vi "2Setpoints.vi"   [LabVIEW 2018]
doc: "The myRIO Project template acquires acceleration data from the onboard accelerometer and displays the changes of acceleration values in a waveform chart."
uses:
  <vilib>/platform/TimedLoop/XDataNode/XDataNode.xnode
  <vilib>/Platform/TimedLoop/XDataNode/nitl_modes.ctl
  <vilib>/Platform/TimedLoop/XDataNode/XDNodeRunTimeDep.lvlib
  <vilib>/Platform/TimedLoop/XDataNode/wakeup.ctl
  <vilib>/Platform/TimedLoop/XDataNode/timing_clust.ctl
  <vilib>/myRIO/Common/Instrument Driver Framework/Utilities/typedefs/Generic FPGA Reference.ctl
  <vilib>/myRIO/Common/Instrument Driver Framework/Utilities/typedefs/myRIO v1.0 Reference.ctl
  <vilib>/myRIO/Common/Instrument Driver Framework/Utilities/typedefs/Hardware Version Enum.ctl
  <vilib>/myRIO/Common/Instrument Driver Framework/Utilities/typedefs/myRIO Generic Hardware Reference.ctl
  <vilib>/userdefined/High Color/nirio_resource_hc.ctl
  <vilib>/myRIO/Common/Instrument Driver Framework/myRIO v1.0/Encoder/typedefs/Encoder Channels Enum.ctl
  <vilib>/myRIO/Instrument Drivers/Onboard IO/Encoder/typedefs/Encoder Reference.ctl
  <vilib>/myRIO/Instrument Drivers/Onboard IO/Encoder/Encoder.lvlib
  <vilib>/myRIO/Common/Instrument Driver Framework/myRIO v1.0/Encoder/typedefs/Encoder Signal Mode.ctl
  <vilib>/myRIO/Instrument Drivers/Onboard IO/Encoder/vis/myRIO Encoder Open.xnode
  <vilib>/myRIO/Common/Instrument Driver Framework/myRIO v1.0/Encoder/vis/myRIO v1.1 Open Encoder.vi
  <vilib>/myRIO/Common/Instrument Driver Framework/myRIO v1.0/Encoder/vis/myRIO v1.0 Configure Encoder.vi
  <vilib>/myRIO/Common/Instrument Driver Framework/myRIO v1.0/Encoder/typedefs/Encoder Configuration v1.0.ctl
  <vilib>/myRIO/Instrument Drivers/Onboard IO/PWM/typedefs/PWM Configuration.ctl
  <vilib>/myRIO/Instrument Drivers/Onboard IO/PWM/PWM.lvlib
  <vilib>/myRIO/Common/Instrument Driver Framework/myRIO v1.0/PWM/typedefs/PWM Channels Enum.ctl
  <vilib>/myRIO/Instrument Drivers/Onboard IO/PWM/typedefs/PWM Reference.ctl
  <vilib>/myRIO/Instrument Drivers/Onboard IO/PWM/vis/myRIO PWM Open.xnode
  <vilib>/myRIO/Common/Instrument Driver Framework/myRIO v1.0/PWM/vis/myRIO v1.1 Open PWM.vi
types:
  T1 = typedef "Encoder Signal Mode.ctl" = enum16{"Quadrature phase signal", "Step and direction signal"}
  T2 = typedef "PWM.lvlib/PWM Reference.ctl" = cluster{"myRIO Reference":T3, "PWM Channels Enum":T7, "PWM Configuration":T8}
  T3 = typedef "myRIO Generic Hardware Reference.ctl" = cluster{"myRIO Model":T4, "myRIO Hardware Reference":T5}
  T4 = typedef "Hardware Version Enum.ctl" = enum16{"Unknown", "myRIO-1900", "myRIO-1950", "roboRIO", "NI ELVIS RIO CM", "ELVIS III"}
  T5 = typedef "myRIO v1.0 Reference.ctl" = cluster{"Generic FPGA Reference":T6, "Allow multiple opens":bool}
  T6 = typedef "Generic FPGA Reference.ctl" = refnum<k20>
  T7 = typedef "PWM Channels Enum.ctl" = enum16{"Not Connected", "C/PWM0", "C/PWM1", "A/PWM0", "A/PWM1", "A/PWM2", "A/PWM3", "A/PWM4", "A/PWM5", "A/PWM6", "A/PWM7", "A/PWM8", "A/PWM9", "A/PWM10", "A/PWM11", "A/PWM12", "A/PWM13", "A/PWM14", "A/PWM15", "A/PWM16", "A/PWM17", "A/PWM18", "A/PWM19", "B/PWM0", "B/PWM1", "B/PWM2", "B/PWM3", "B/PWM4", "B/PWM5", "B/PWM6", "B/PWM7", "B/PWM8", "B/PWM9", "B/PWM10", "B/PWM11", "B/PWM12", "B/PWM13", "B/PWM14", "B/PWM15", "B/PWM16", "B/PWM17", "B/PWM18", "B/PWM19", "PWM/PWM0", "PWM/PWM1", "PWM/PWM2", "PWM/PWM3", "PWM/PWM4", "PWM/PWM5", "PWM/PWM6", "PWM/PWM7", "PWM/PWM8", "PWM/PWM9"}
  T8 = typedef "PWM.lvlib/PWM Configuration.ctl" = cluster{"Frequency":dbl, "Duty Cycle":dbl}
  T9 = typedef "Encoder.lvlib/Encoder Reference.ctl" = cluster{"myRIO Reference":T3, "Encoder Channels Enum":T10}
  T10 = typedef "Encoder Channels Enum.ctl" = enum16{"Not Connected", "C/ENC0", "C/ENC1", "A/ENC", "A/ENC0", "A/ENC1", "A/ENC2", "A/ENC3", "A/ENC4", "A/ENC5", "A/ENC6", "A/ENC7", "A/ENC8", "A/ENC9", "B/ENC", "B/ENC0", "B/ENC1", "B/ENC2", "B/ENC3", "B/ENC4", "B/ENC5", "B/ENC6", "B/ENC7", "B/ENC8", "B/ENC9", "DIO/ENC0", "DIO/ENC1", "DIO/ENC2", "DIO/ENC3", "DIO/ENC4"}
  T11 = typedef "XDNodeRunTimeDep.lvlib/timing_clust.ctl" = cluster{"Expected End [f-1]":u64, "Actual End [f-1]":u64, "Finished Late? [f-1]":bool, "Expected End [i-1]":u64, "Actual End [i-1]":u64, "Finished Late? [i-1]":bool, "Expected Start [i]":u64, "Actual Start [i]":u64, "Expected Start [f]":u64, "Actual Start [f]":u64, "Source Name":string, "Structure Name":string, "Period":i64, "Deadline":i64, "Offset":i64, "Start":i64, "Priority":i32, "Timeout":i32, "Mode":T12, "Wakeup Reason":T13, "Error":errorcluster, "Source Type":string, "Secondary Source Type":string, "Global End Time":u64, "Global Start Time":u64, "Frame Duration":u64, "Iteration Duration":u64, "Assigned CPU":i32, "I/O Scan Engine Mode":u32}
  T12 = typedef "XDNodeRunTimeDep.lvlib/nitl_modes.ctl" = enum32{"No Change", "Process missed periods, maintain original phase", "Discard missed periods, maintain original phase", "Process missed periods, ignore original phase", "Discard missed periods, ignore original phase"}
  T13 = typedef "XDNodeRunTimeDep.lvlib/wakeup.ctl" = enum32{"Normal", "Aborted", "Asynchronous wakeup", "Timing source error", "Timed loop error", "Timeout"}
  T14 = cluster{"Double":dbl, dbl, dbl, "seconds since 1Jan1904":timestamp, "Double":dbl, dbl, dbl}
  T15 = cluster{"Double":dbl, "dbl Scaled Value":dbl, "Output":dbl, "seconds since 1Jan1904":timestamp, dbl, dbl, dbl}
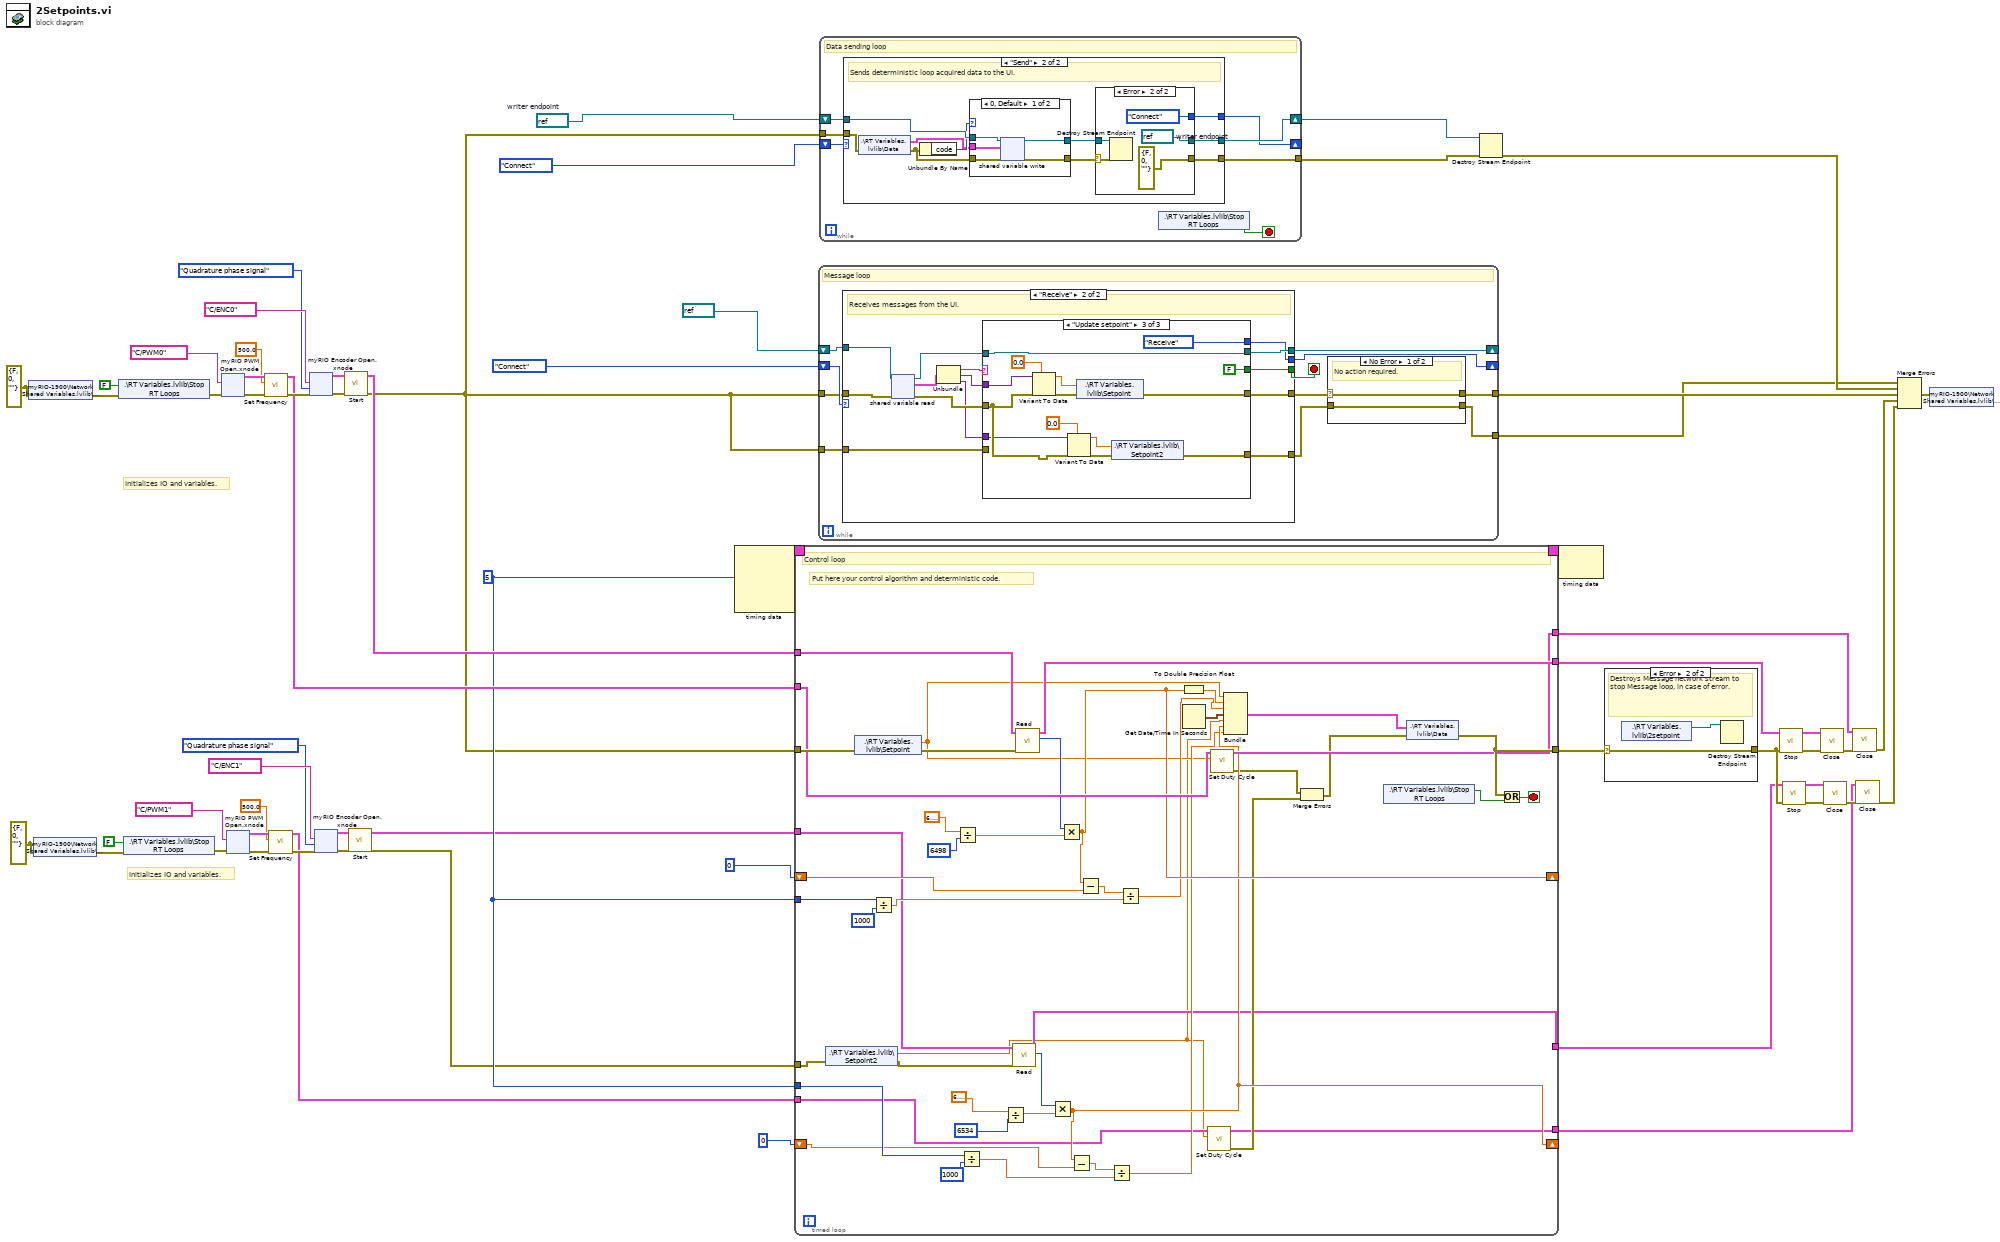
[diagram p0: block diagram]
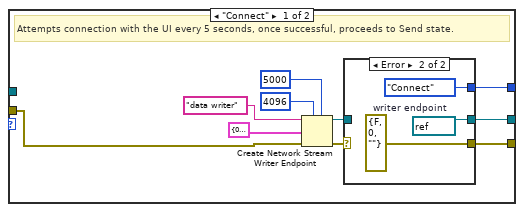
[diagram p3: hidden frame]
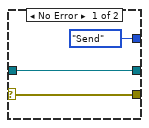
[diagram p4: hidden frame]
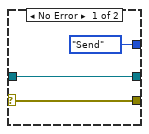
[diagram p5: hidden frame]
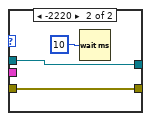
[diagram p6: hidden frame]
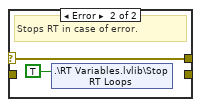
[diagram p7: hidden frame]
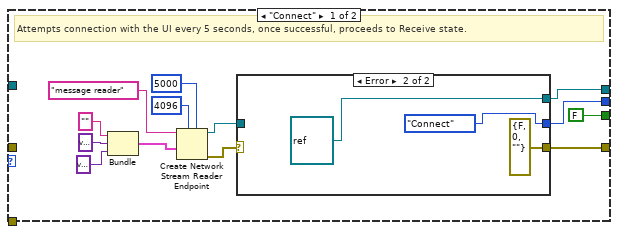
[diagram p8: hidden frame]
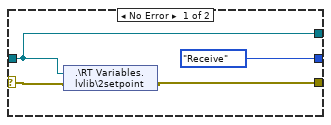
[diagram p9: hidden frame]
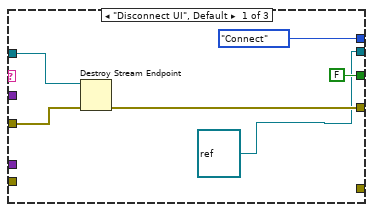
[diagram p10: hidden frame]
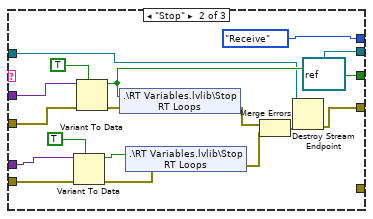
[diagram p11: hidden frame]
diagram:
  w11 = refnum<k21> refnum  # writer endpoint
  w26 = errorcluster {"status"=FALSE, "code"=0, "source"=""} ("error IO")
  w29 = i64 5 ("Period")
  w50 = errorcluster {"status"=FALSE, "code"=0, "source"=""} ("error IO")
  # "Initializes IO and variables."
  # "Initializes IO and variables."
  n1 = shared-variable "myRIO-1900\\Network Shared Variables.lvlib\\error IO"(w50, error in=w50) -> (error out=w51:errorcluster)
  n2 = shared-variable "myRIO-1900\\Network Shared Variables.lvlib\\error IO"(w26, error in=w26) -> (error out=w27:errorcluster)
  n3 = shared-variable ".\\RT Variables.lvlib\\Stop RT Loops"(FALSE ("Stop RT Loops"), error in=w51) -> (error out=w38:errorcluster)
  n4 = shared-variable ".\\RT Variables.lvlib\\Stop RT Loops"(FALSE ("Stop RT Loops"), error in=w27) -> (error out=w19:errorcluster)
  n5 = xnode "myRIO PWM Open.xnode"("error in (no error)"=w38, "Channel Name"=tag "C/PWM0") -> ("error out"=w40:errorcluster, "PWM Ref Out"=w39:T2)  [unwired: 1 in]
  n6 = xnode "myRIO PWM Open.xnode"("error in (no error)"=w19, "Channel Name"=tag "C/PWM1") -> ("error out"=w21:errorcluster, "PWM Ref Out"=w20:T2)  [unwired: 1 in]
  n7 = call <vilib>:"Set Frequency.vi"("error in (no error)"=w40, "Frequency [Hz]"=500.0, "PWM Ref In"=w39) -> ("error out"=w37:errorcluster, "PWM Ref Out"=w34:T2)  [unwired: 6 in]
  n8 = call <vilib>:"Set Frequency.vi"("error in (no error)"=w21, "Frequency [Hz]"=500.0, "PWM Ref In"=w20) -> ("error out"=w18:errorcluster, "PWM Ref Out"=w13:T2)  [unwired: 6 in]
  n9 = xnode "myRIO Encoder Open.xnode"("error in (no error)"=w37, "Channel Name"=tag "C/ENC0", "Encoder Signal Mode"=Encoder_Signal_Mode."Quadrature phase signal") -> ("error out"=w47:errorcluster, "Encoder Ref Out"=w46:T9)  [unwired: 2 in]
  n10 = xnode "myRIO Encoder Open.xnode"("error in (no error)"=w18, "Channel Name"=tag "C/ENC1", "Encoder Signal Mode"=Encoder_Signal_Mode."Quadrature phase signal") -> ("error out"=w24:errorcluster, "Encoder Ref Out"=w23:T9)  [unwired: 2 in]
  n11 = call <vilib>:"Start.vi"("error in (no error)"=w47, "Encoder Ref In"=w46) -> ("error out"=w1:errorcluster, "Encoder Ref Out"=w44:T9)  [unwired: 8 in]
  n12 = call <vilib>:"Start.vi"("error in (no error)"=w24, "Encoder Ref In"=w23) -> ("error out"=w15:errorcluster, "Encoder Ref Out"=w14:T9)  [unwired: 8 in]
  n13 = node-c288(w29) -> (w61:T11)  [unwired: 3 in]
  n14 = timed-loop {
    timing: w61 -> [_]
    timing-out: [_] -> w60
    tunnel: w1 -> [w105]
    tunnel: [w101] -> w49
    tunnel: w44 -> [w100]
    tunnel: [w99] -> w41
    tunnel: w34 -> [w98]
    tunnel: [w96] -> w33
    shift-right: [w90] -> _
    shift-left: 0 -> [w89]
    tunnel: w29 -> [w86]
    shift-right: [w73] -> _
    shift-left: 0 -> [w78]
    tunnel: w29 -> [w79]
    tunnel: w15 -> [w64]
    tunnel: w14 -> [w75]
    tunnel: w13 -> [w71]
    tunnel: [w66] -> w6
    tunnel: [w65] -> w5
    stop <- w102 stop-if-true
    # "Put here your control algorithm and deterministic code."
    # "Control loop"
    n15 = shared-variable ".\\RT Variables.lvlib\\Setpoint2"(error in=w64) -> (w62:dbl, error out=w63:errorcluster)
    n16 = shared-variable ".\\RT Variables.lvlib\\Setpoint"(error in=w105) -> (w67:dbl, error out=w106:errorcluster)
    n17 = Divide(x=w86, y=1000) -> (x/y=w84:dbl)
    n18 = Divide(x=6.283185307179586, y=6498) -> (x/y=w91:dbl)
    n19 = Divide(x=w79, y=1000) -> (x/y=w74:dbl)
    n20 = Divide(x=6.283185307179586, y=6534) -> (x/y=w76:dbl)
    n21 = call <vilib>:"Read.vi"("error in (no error)"=w63, "Encoder Ref In"=w75) -> ("Counter Value"=w77:i32, "Encoder Ref Out"=w66:T9)  [unwired: 5 in, 3 out]
    n22 = call <vilib>:"Read.vi"("error in (no error)"=w106, "Encoder Ref In"=w100) -> ("Counter Value"=w92:i32, "Encoder Ref Out"=w99:T9)  [unwired: 5 in, 3 out]
    n23 = Multiply(x=w77, y=w76) -> (x*y=w73:dbl)
    n24 = Multiply(x=w92, y=w91) -> (x*y=w90:dbl)
    n25 = Subtract(x=w73, y=w78) -> (x-y=w80:dbl)
    n26 = Subtract(x=w90, y=w89) -> (x-y=w88:dbl)
    n27 = Divide(x=w80, y=w74) -> (x/y=w72:dbl)
    n28 = Divide(x=w88, y=w84) -> (x/y=w87:dbl)
    n29 = To Double Precision Float(number=w90) -> (double precision float=w97:dbl)
    n30 = Get Date/Time In Seconds() -> (seconds since 1Jan1904=w104:timestamp)
    n31 = call <vilib>:"Set Duty Cycle.vi"("Duty Cycle"=w62, "PWM Ref In"=w71) -> ("error out"=w70:errorcluster, "PWM Ref Out"=w65:T2)  [unwired: 7 in]
    n32 = call <vilib>:"Set Duty Cycle.vi"("Duty Cycle"=w67, "PWM Ref In"=w98) -> ("error out"=w69:errorcluster, "PWM Ref Out"=w96:T2)  [unwired: 7 in]
    n33 = Bundle("Double"=w67, w97, w87, "seconds since 1Jan1904"=w104, "Double"=w62, w73, w72) -> (w95:T14)  [unwired: 1 in]
    n34 = Merge Errors(w69, w70) -> (w68:errorcluster)
    n35 = shared-variable ".\\RT Variables.lvlib\\Stop RT Loops"() -> (w103:bool)  [unwired: 1 in, 1 out]
    n36 = shared-variable ".\\RT Variables.lvlib\\Data"(w95, error in=w68) -> (error out=w101:errorcluster)
    n37 = Or(x=w101, y=w103) -> (x .or. y?=w102:bool)
  }
  n38 = while {
    tunnel: [w113] -> w53
    shift-right: [w118] -> _
    shift-left: refnum<k21> refnum ("reader endpoint") -> [w116]
    shift-right: [w117] -> _
    shift-left: enum16{"Connect", "Receive"}."Connect" ("Message states") -> [w119]
    tunnel: w1 -> [w115]
    tunnel: [w111] -> w3
    tunnel: w1 -> [w109]
    stop <- w110 stop-if-true
    # "Message loop"
    n39 = case shown="\"Receive\"" w119 {
      tunnel: [w127 w153] -> w114
      tunnel: [w125 w154] -> w118
      tunnel: [w134 w150] -> w117
      tunnel: w116 -> [_ w148]
      tunnel: w115 -> [_ w152]
      tunnel: [FALSE ("Stop RT Loops") w151] -> w110
      tunnel: [_ w145] -> w112
      tunnel: w109 -> [_ w144]
      frame "Connect" {
        # "Attempts connection with the UI every 5 seconds, once successful, proceeds to Receive state."
        n40 = Bundle("", variant, variant) -> (w130:cluster{string, variant, variant})  [unwired: 1 in]
        n41 = Create Network Stream Reader Endpoint(5:5000 ("timeout in ms (-1)"), 7:4096 ("reader buffer size"), 9:w130, 11:"message reader" ("reader name")) -> (0:w129:errorcluster, 3:w124:refnum<k21>)  [unwired: 3 in]
        n42 = case shown="Error" w129 {
          selector: w129 -> [w138 _]
          tunnel: [enum16{"Connect", "Receive"}."Receive" ("Message states") enum16{"Connect", "Receive"}."Connect" ("Message states")] -> w134
          tunnel: [w137 errorcluster {"status"=FALSE, "code"=0, "source"=""} ("error IO")] -> w127
          tunnel: [w139 refnum<k21> refnum ("reader endpoint")] -> w125
          tunnel: w124 -> [w139 _]
          frame No Error {
            n43 = shared-variable ".\\RT Variables.lvlib\\2setpoint"(w139, error in=w138) -> (error out=w137:errorcluster)
          }
          frame Error {
          }
        }
      }
      frame "Receive" {
        # "Receives messages from the UI."
        n44 = shared-variable-read(w148, w152) -> (w147:refnum<k21>, w155:errorcluster, w149:cluster{string, variant, variant})  [unwired: 1 in, 1 out]
        n45 = Unbundle(w149) -> (w157:string, w156:variant, w146:variant)
        n46 = case shown="\"Update setpoint\"" w157 {
          tunnel: w156 -> [_ w178 w194]
          tunnel: w155 -> [w161 w180 w183]
          tunnel: [w160 w175 w190] -> w153
          tunnel: [refnum<k21> refnum ("reader endpoint") refnum<k21> refnum ("reader endpoint") w189] -> w154
          tunnel: w147 -> [w159 w174 w189]
          tunnel: [FALSE ("Stop RT Loops") w177 FALSE ("Stop RT Loops")] -> w151
          tunnel: [enum16{"Connect", "Receive"}."Connect" ("Message states") enum16{"Connect", "Receive"}."Receive" ("Message states") enum16{"Connect", "Receive"}."Receive" ("Message states")] -> w150
          tunnel: w146 -> [_ w170 w182]
          tunnel: [_ _ w181] -> w145
          tunnel: w144 -> [_ w169 _]
          frame "Disconnect UI", Default {
            n47 = Destroy Stream Endpoint(8:w161, 11:w159) -> (0:w160:errorcluster)
          }
          frame "Stop" {
            n48 = Variant To Data(error in=w169, type=TRUE ("Stop RT Loops"), Variant=w170) -> (data=w167:bool, error out=w171:errorcluster)
            n49 = Variant To Data(error in=w180, type=TRUE ("Stop RT Loops"), Variant=w178) -> (data=w177:bool, error out=w179:errorcluster)
            n50 = shared-variable ".\\RT Variables.lvlib\\Stop RT Loops"(w177, error in=w179) -> (error out=w165:errorcluster)
            n51 = shared-variable ".\\RT Variables.lvlib\\Stop RT Loops"(w167, error in=w171) -> (error out=w166:errorcluster)
            n52 = Merge Errors(w165, w166) -> (w164:errorcluster)
            n53 = Destroy Stream Endpoint(8:w164, 11:w174) -> (0:w175:errorcluster)
          }
          frame "Update setpoint" {
            n54 = Variant To Data(error in=w183, type=0.0, Variant=w194) -> (data=w192:dbl, error out=w191:errorcluster)
            n55 = Variant To Data(error in=w183, type=0.0, Variant=w182) -> (data=w185:dbl, error out=w184:errorcluster)
            n56 = shared-variable ".\\RT Variables.lvlib\\Setpoint"(w192, error in=w191) -> (error out=w190:errorcluster)
            n57 = shared-variable ".\\RT Variables.lvlib\\Setpoint2"(w185, error in=w184) -> (error out=w181:errorcluster)
          }
        }
      }
    }
    n58 = case shown="No Error" w114 {
      selector: w114 -> [w121 w122]
      tunnel: [w121 w122] -> w113
      tunnel: w112 -> [w120 _]
      tunnel: [w120 _] -> w111
      frame No Error {
        # "No action required."
      }
      frame Error {
        # "Stops RT in case of error."
        n59 = shared-variable ".\\RT Variables.lvlib\\Stop RT Loops"(TRUE ("Stop RT Loops")) -> ()  [unwired: 1 in, 1 out]
      }
    }
  }
  n60 = while {
    shift-right: [w199] -> w56
    shift-left: w11 -> [w197]
    tunnel: [w198] -> w57
    tunnel: w1 -> [w196]
    shift-right: [w195] -> _
    shift-left: enum16{"Connect", "Send"}."Connect" ("Message states") -> [w200]
    stop <- w201 stop-if-true
    # "Data sending loop"
    n61 = case shown="\"Send\"" w200 {
      tunnel: [w205 w220] -> w198
      tunnel: [w203 w218] -> w199
      tunnel: [w209 w221] -> w195
      tunnel: w197 -> [_ w227]
      tunnel: w196 -> [w206 w226]
      frame "Connect" {
        # "Attempts connection with the UI every 5 seconds, once successful, proceeds to Send state."
        n62 = Create Network Stream Writer Endpoint(5:5000 ("timeout in ms (-1)"), 7:4096 ("writer buffer size"), 8:w206, 9:T15 {"Double"=0.0, "dbl Scaled Value"=0.0, "Output"=0.0, "seconds since 1Jan1904"=timestamp(0 s since 1904-01-01), 0.0, 0.0, 0.0} ("Data"), 11:"data writer" ("writer name")) -> (0:w207:errorcluster, 3:w204:refnum<k21>)  [unwired: 2 in]
        n63 = case shown="Error" w207 {
          selector: w207 -> [w212 _]
          tunnel: [enum16{"Connect", "Send"}."Send" ("Message states") enum16{"Connect", "Send"}."Connect" ("Message states")] -> w209
          tunnel: [w212 errorcluster {"status"=FALSE, "code"=0, "source"=""} ("error IO")] -> w205
          tunnel: w204 -> [w214 _]
          tunnel: [w214 w215] -> w203
          frame No Error {
          }
          frame Error {
            w215 = refnum<k21> refnum  # writer endpoint
          }
        }
      }
      frame "Send" {
        # "Sends deterministic loop acquired data to the UI."
        n64 = shared-variable ".\\RT Variables.lvlib\\Data"(error in=w226) -> (w223:T15, error out=w225:errorcluster)
        n65 = Unbundle By Name(w225) -> ("code"=w224:i32)
        n66 = case shown="0, Default" w224 {
          tunnel: [w240 w242] -> w222
          tunnel: [w239 w241] -> w219
          tunnel: w227 -> [w238 w241]
          tunnel: w225 -> [w237 w242]
          tunnel: w223 -> [w236 _]
          frame 0, Default {
            n67 = shared-variable-write(w238, w237, w236) -> (w239:refnum<k21>, w240:errorcluster)  [unwired: 1 in, 1 out]
          }
          frame -2220 {
            n68 = Wait (ms)(milliseconds to wait=u32 10) -> ()  [unwired: 1 out]
          }
        }
        n69 = case shown="Error" w222 {
          selector: w222 -> [w230 w234]
          tunnel: [enum16{"Connect", "Send"}."Send" ("Message states") enum16{"Connect", "Send"}."Connect" ("Message states")] -> w221
          tunnel: [w230 errorcluster {"status"=FALSE, "code"=0, "source"=""} ("error IO")] -> w220
          tunnel: w219 -> [w228 w233]
          tunnel: [w228 w231] -> w218
          frame No Error {
          }
          frame Error {
            w231 = refnum<k21> refnum  # writer endpoint
            n70 = Destroy Stream Endpoint(8:w234, 11:w233) -> ()  [unwired: 1 out]
          }
        }
      }
    }
    n71 = shared-variable ".\\RT Variables.lvlib\\Stop RT Loops"() -> (w201:bool)  [unwired: 1 in, 1 out]
  }
  n72 = Destroy Stream Endpoint(8:w57, 11:w56) -> (0:w54:errorcluster)
  n73 = node-c288(w60) -> ()  [unwired: 1 out]
  n74 = case shown="Error" w49 {
    selector: w49 -> [w244 w245]
    tunnel: [w244 w245] -> w7
    frame No Error {
      # "No action required."
    }
    frame Error {
      # "Destroys Message network stream to stop Message loop, in case of error."
      n75 = shared-variable ".\\RT Variables.lvlib\\2setpoint"() -> (w246:refnum<k21>)  [unwired: 1 in, 1 out]
      n76 = Destroy Stream Endpoint(11:w246) -> ()  [unwired: 1 in, 1 out]
    }
  }
  n77 = call <vilib>:"Stop.vi"("error in (no error)"=w7, "Encoder Ref In"=w41) -> ("error out"=w42:errorcluster, "Encoder Ref Out"=w43:T9)  [unwired: 8 in]
  n78 = call <vilib>:"Stop.vi"("error in (no error)"=w7, "Encoder Ref In"=w6) -> ("error out"=w9:errorcluster, "Encoder Ref Out"=w10:T9)  [unwired: 8 in]
  n79 = call <vilib>:"Close.vi"("error in (no error)"=w42, "Encoder Ref In"=w43) -> ("error out"=w36:errorcluster)  [unwired: 9 in]
  n80 = call <vilib>:"Close.vi"("error in (no error)"=w9, "Encoder Ref In"=w10) -> ("error out"=w8:errorcluster)  [unwired: 9 in]
  n81 = call <vilib>:"Close.vi"("error in (no error)"=w36, "PWM Ref In"=w33) -> ("error out"=w35:errorcluster)  [unwired: 9 in]
  n82 = call <vilib>:"Close.vi"("error in (no error)"=w8, "PWM Ref In"=w5) -> ("error out"=w4:errorcluster)  [unwired: 9 in]
  n83 = Merge Errors(w3, w54, w53, w35, w4) -> (w52:errorcluster)
  n84 = shared-variable "myRIO-1900\\Network Shared Variables.lvlib\\error IO"(w52) -> ()  [unwired: 1 in, 1 out]
